vi "5.3 2D-Cluster to CSM API String.vi"() -> ()   [LabVIEW 2017]
uses:
  9f1c8977-aa41-4596-a18a-6dba2ebc59d2.vi
  0333efe5-f0fb-4901-b6dd-db031cec30c6.vi
  addons/API-String-Arugments-Support/_Support/Data To API String Arguments.vi
  addons/API-String-Arugments-Support/_Support/Convert API String Arguments to Data(variant).vi
panel:
  out "String":string
  in  "Array":T1(array[cluster])=[[{"String"="abc", "BoolArray"=[[TRUE, FALSE, TRUE, FALSE], [FALSE, TRUE, FALSE, TRUE], [TRUE, FALSE, TRUE, FALSE]], "Boolean"=FALSE}, {"String"="def", "BoolArray"=[[TRUE, FALSE, TRUE, FALSE], [FALSE, TRUE, FALSE, TRUE], [TRUE, FALSE, TRUE, FALSE]], "Boolean"=TRUE}], [{"String"="123", "BoolArray"=[[FALSE, FALSE, TRUE, FALSE], [FALSE, TRUE, FALSE, TRUE], [TRUE, TRUE, TRUE, FALSE]], "Boolean"=TRUE}, {"String"="456", "BoolArray"=[[TRUE, TRUE, TRUE, FALSE], [TRUE, FALSE, FALSE, TRUE], [FALSE, FALSE, TRUE, FALSE]], "Boolean"=FALSE}]]
  out "Array":T1(array[cluster])=[[{"String"="abc", "BoolArray"=[[TRUE, FALSE, TRUE, FALSE], [FALSE, TRUE, FALSE, TRUE], [TRUE, FALSE, TRUE, FALSE]], "Boolean"=FALSE}, {"String"="def", "BoolArray"=[[TRUE, FALSE, TRUE, FALSE], [FALSE, TRUE, FALSE, TRUE], [TRUE, FALSE, TRUE, FALSE]], "Boolean"=TRUE}]]
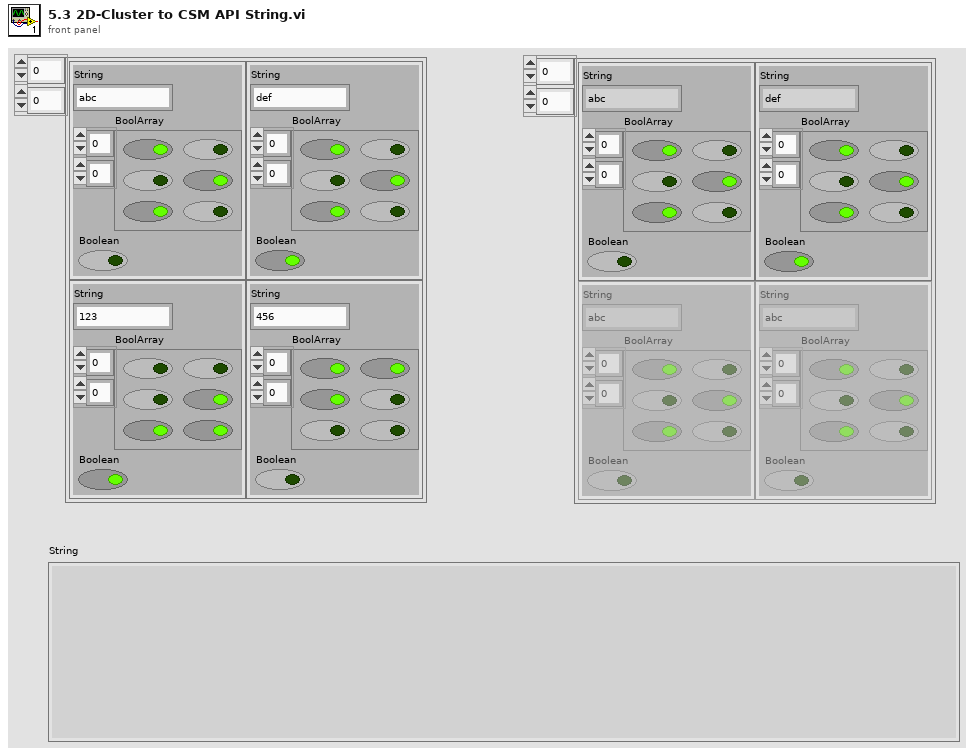
[diagram p1: front panel]
types:
  T1 = cluster{"String":string, "BoolArray":bool[][], "Boolean":bool}[][]
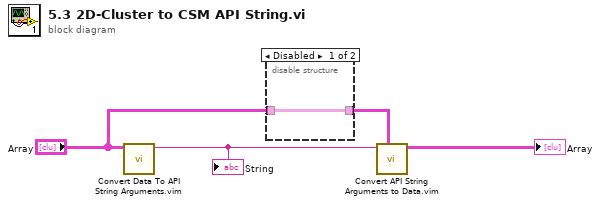
[diagram p0: block diagram]
diagram:
  n1 = call "Convert Data To API String Arguments.vim"("data"="Array") -> ("String"=w1:string)  [unwired: 7 in, 1 out]
  "String" <- w1
  n2 = disable-structure "Diagram Disable Structure" shown="Disabled" {
    disable-tunnel: "Array" -> [w5 _]
    disable-tunnel: [w5 _] -> w3
    frame Disabled {
    }
    frame Enabled {
    }
  }
  n3 = call "Convert API String Arguments to Data.vim"("Type"=w3, "String"=w1) -> ("Data"=→"Array":T1)  [unwired: 6 in, 1 out]
